vi "Simulation.vi"() -> ()   [LabVIEW 2011]
uses:
  Pumps_Valves_Dependencies_Global.vi
panel:
  out "Slide":dbl(slide) scale=0.0..100.0
  out "Supply feed  2":bool(c317)
  out "Pipe3":bool
  out "T-Pipe 2":bool
  out "Supply feed  2":bool(c317)
  out "Pipe5":bool
  out "Pipe4":bool
  out "Mains Water Supply":bool
  out "Pipe2":bool
  out "Supply feed":bool(c317)
  out "T-Pipe":bool
  out "Tank C":dbl(slide) scale=0.0..100.0
  out "Tank D":dbl(slide) scale=0.0..100.0
  out "Tank B":dbl(slide) scale=0.0..100.0
  out "Pipe":bool
  out "Pipe 1":bool
  out "Tank A":dbl(slide) scale=0.0..100.0
  out "Salt Saturator":dbl(slide) scale=0.0..100.0
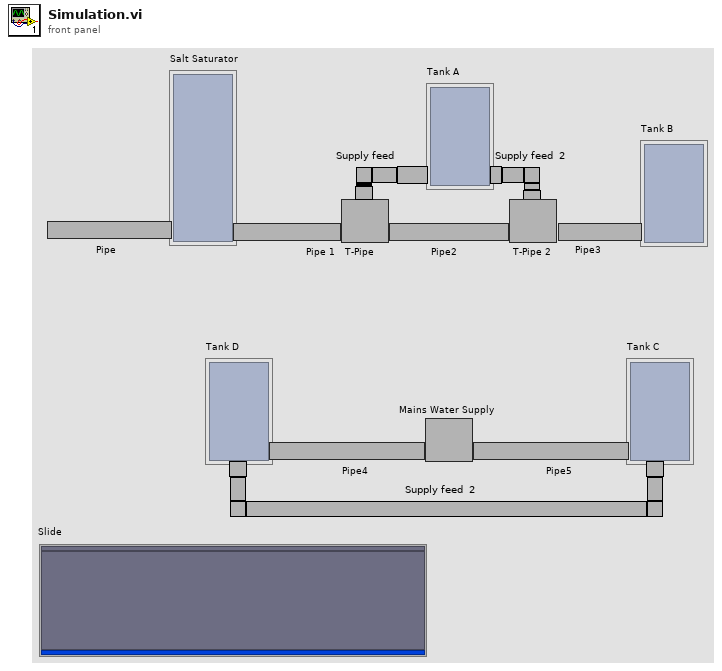
[diagram p1: front panel]
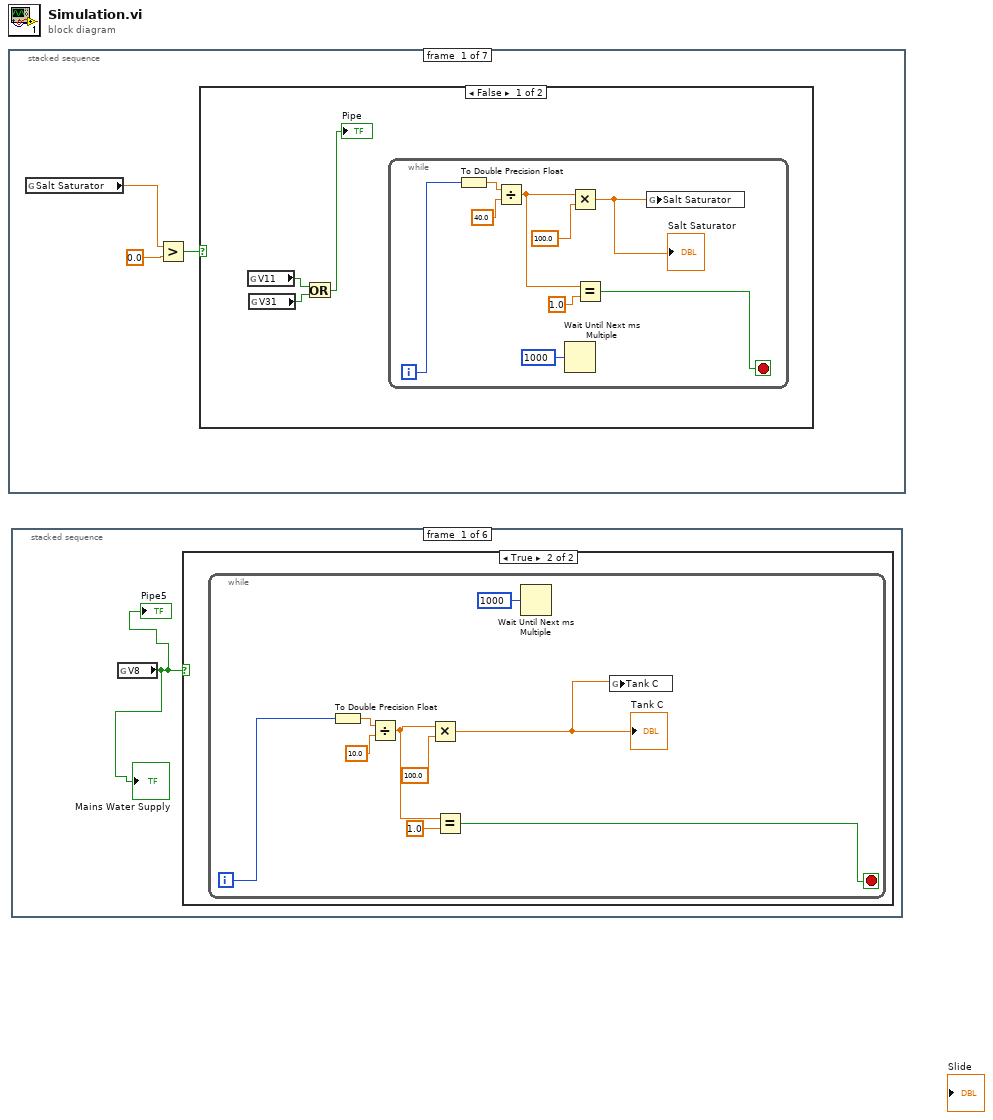
[diagram p0: block diagram]
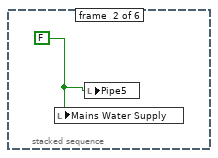
[diagram p3: hidden frame]
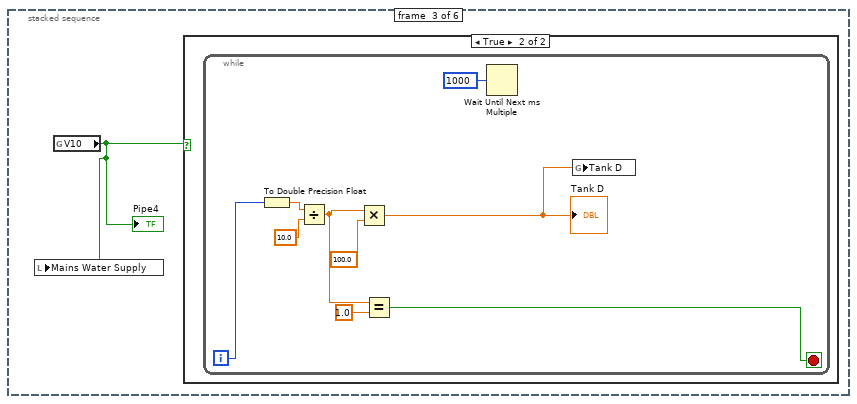
[diagram p4: hidden frame]
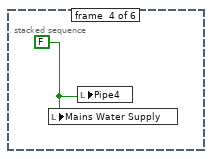
[diagram p6: hidden frame]
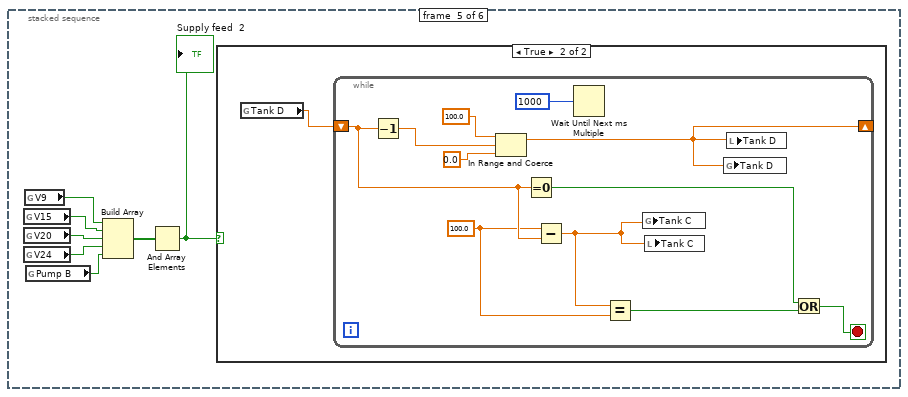
[diagram p7: hidden frame]
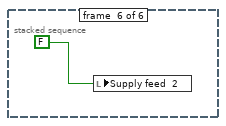
[diagram p9: hidden frame]
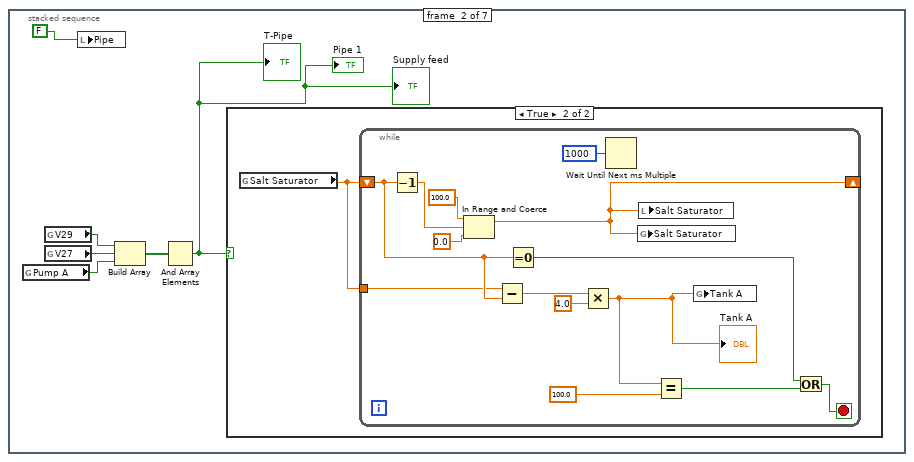
[diagram p11: hidden frame]
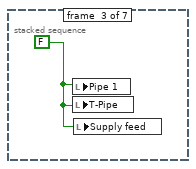
[diagram p13: hidden frame]
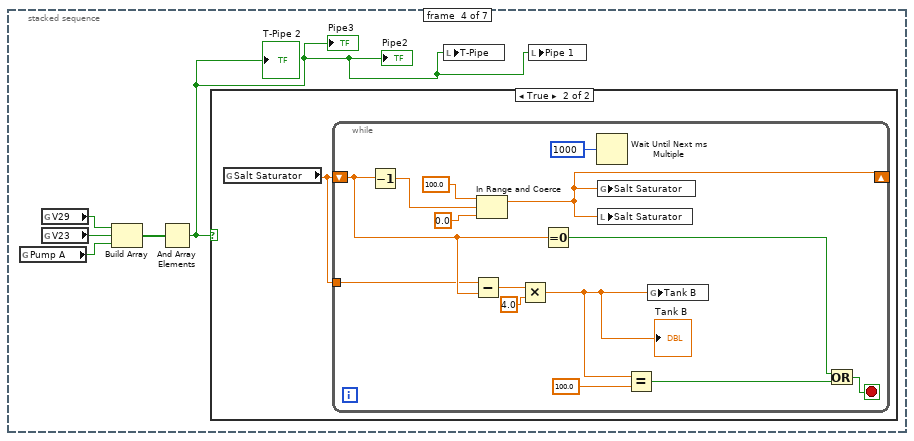
[diagram p14: hidden frame]
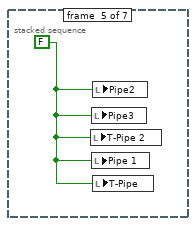
[diagram p16: hidden frame]
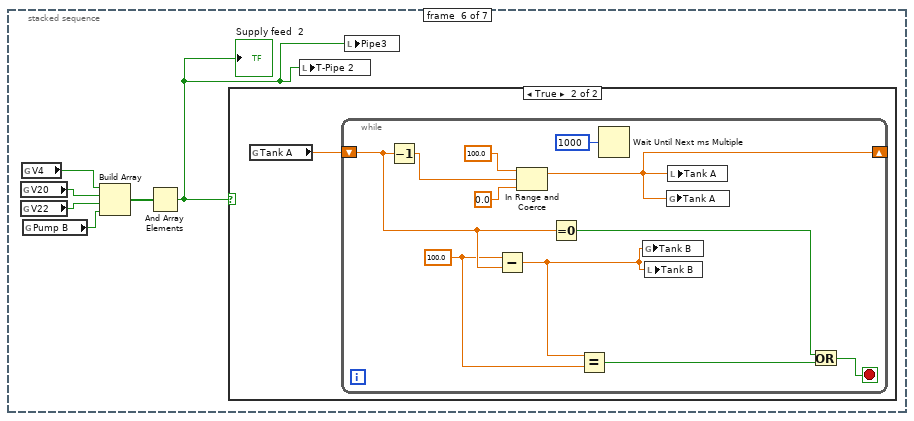
[diagram p17: hidden frame]
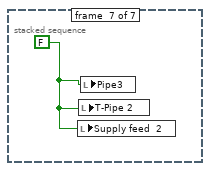
[diagram p19: hidden frame]
diagram:
  n1 = stacked-sequence {
    frame #0 {
      n2 = global read "Pumps_Valves_Dependencies_Global.vi" "Salt Saturator"() -> (w2:dbl)
      n3 = Greater?(x=w2, y=0.0) -> (0:w3:bool)
      n4 = case shown="False" w3 {
        frame False {
          n5 = global read "Pumps_Valves_Dependencies_Global.vi" "V11"() -> (w5:bool)
          n6 = global read "Pumps_Valves_Dependencies_Global.vi" "V31"() -> (w6:bool)
          n7 = Or(x=w5, y=w6) -> (x .or. y?=→"Pipe":bool)
          n8 = while {
            i -> [w7]
            stop <- w9 stop-if-true
            n9 = To Double Precision Float(number=w7) -> (double precision float=w11:dbl)
            n10 = Divide(x=w11, y=40.0) -> (x/y=w13:dbl)
            n11 = Wait Until Next ms Multiple(millisecond multiple=u32 1000) -> ()  [unwired: 1 out]
            n12 = Multiply(x=w13, y=100.0) -> (x*y=w8:dbl)
            "Salt Saturator" <- w8
            n13 = Equal?(x=w13, y=1.0) -> (x = y?=w9:bool)
            n14 = global write "Pumps_Valves_Dependencies_Global.vi" "Salt Saturator"(w8) -> ()
          }
        }
        frame True {
        }
      }
    }
    frame #1 {
      n15 = global read "Pumps_Valves_Dependencies_Global.vi" "Pump A"() -> (w19:bool)
      n16 = global read "Pumps_Valves_Dependencies_Global.vi" "V29"() -> (w17:bool)
      n17 = global read "Pumps_Valves_Dependencies_Global.vi" "V27"() -> (w18:bool)
      n18 = local write "Pipe"(FALSE) -> ()
      n19 = Build Array(w17, w18, w19) -> (w20:bool[])
      n20 = And Array Elements(Boolean array=w20) -> (logical AND=w16:bool)
      "Pipe 1" <- w16
      "T-Pipe" <- w16
      "Supply feed" <- w16
      n21 = case shown="True" w16 {
        frame False {
        }
        frame True {
          n22 = global read "Pumps_Valves_Dependencies_Global.vi" "Salt Saturator"() -> (w22:dbl)
          n23 = while {
            shift-right: [w30] -> _
            shift-left: w22 -> [w26]
            tunnel: w22 -> [w23]
            stop <- w34 stop-if-true
            n24 = Decrement(x=w26) -> (x-1=w31:dbl)
            n25 = In Range and Coerce(upper limit=100.0 ("x"), x=w31, lower limit=0.0 ("x")) -> (coerced(x)=w30:dbl)  [unwired: 1 out]
            n26 = Subtract(x=w23, y=w26) -> (x-y=w27:dbl)
            n27 = Equal To 0?(x=w26) -> (x = 0?=w35:bool)
            n28 = Multiply(x=w27, y=4.0) -> (x*y=w24:dbl)
            "Tank A" <- w24
            n29 = Wait Until Next ms Multiple(millisecond multiple=u32 1000) -> ()  [unwired: 1 out]
            n30 = global write "Pumps_Valves_Dependencies_Global.vi" "Salt Saturator"(w30) -> ()
            n31 = local write "Salt Saturator"(w30) -> ()
            n32 = Equal?(x=w24, y=100.0) -> (x = y?=w29:bool)
            n33 = global write "Pumps_Valves_Dependencies_Global.vi" "Tank A"(w24) -> ()
            n34 = Or(x=w35, y=w29) -> (x .or. y?=w34:bool)
          }
        }
      }
    }
    frame #2 {
      w37 = FALSE
      n35 = local write "Pipe 1"(w37) -> ()
      n36 = local write "T-Pipe"(w37) -> ()
      n37 = local write "Supply feed"(w37) -> ()
    }
    frame #3 {
      n38 = global read "Pumps_Valves_Dependencies_Global.vi" "Pump A"() -> (w41:bool)
      n39 = global read "Pumps_Valves_Dependencies_Global.vi" "V29"() -> (w39:bool)
      n40 = global read "Pumps_Valves_Dependencies_Global.vi" "V23"() -> (w40:bool)
      n41 = Build Array(w39, w40, w41) -> (w42:bool[])
      n42 = And Array Elements(Boolean array=w42) -> (logical AND=w38:bool)
      "Pipe2" <- w38
      "T-Pipe 2" <- w38
      "Pipe3" <- w38
      n43 = case shown="True" w38 {
        frame False {
        }
        frame True {
          n44 = global read "Pumps_Valves_Dependencies_Global.vi" "Salt Saturator"() -> (w43:dbl)
          n45 = while {
            shift-right: [w52] -> _
            shift-left: w43 -> [w49]
            tunnel: w43 -> [w45]
            stop <- w55 stop-if-true
            n46 = Decrement(x=w49) -> (x-1=w51:dbl)
            n47 = Subtract(x=w45, y=w49) -> (x-y=w47:dbl)
            n48 = In Range and Coerce(upper limit=100.0 ("x"), x=w51, lower limit=0.0 ("x")) -> (coerced(x)=w52:dbl)  [unwired: 1 out]
            n49 = Multiply(x=w47, y=4.0) -> (x*y=w46:dbl)
            "Tank B" <- w46
            n50 = Equal To 0?(x=w49) -> (x = 0?=w56:bool)
            n51 = Wait Until Next ms Multiple(millisecond multiple=u32 1000) -> ()  [unwired: 1 out]
            n52 = global write "Pumps_Valves_Dependencies_Global.vi" "Salt Saturator"(w52) -> ()
            n53 = local write "Salt Saturator"(w52) -> ()
            n54 = Equal?(x=w46, y=100.0 ("x")) -> (x = y?=w50:bool)
            n55 = global write "Pumps_Valves_Dependencies_Global.vi" "Tank B"(w46) -> ()
            n56 = Or(x=w56, y=w50) -> (x .or. y?=w55:bool)
          }
        }
      }
      n57 = local write "T-Pipe"(w38) -> ()
      n58 = local write "Pipe 1"(w38) -> ()
    }
    frame #4 {
      w58 = FALSE
      n59 = local write "T-Pipe 2"(w58) -> ()
      n60 = local write "Pipe3"(w58) -> ()
      n61 = local write "Pipe 1"(w58) -> ()
      n62 = local write "Pipe2"(w58) -> ()
      n63 = local write "T-Pipe"(w58) -> ()
    }
    frame #5 {
      n64 = global read "Pumps_Valves_Dependencies_Global.vi" "V20"() -> (w63:bool)
      n65 = global read "Pumps_Valves_Dependencies_Global.vi" "V22"() -> (w62:bool)
      n66 = global read "Pumps_Valves_Dependencies_Global.vi" "V4"() -> (w64:bool)
      n67 = global read "Pumps_Valves_Dependencies_Global.vi" "Pump B"() -> (w61:bool)
      n68 = Build Array(w64, w63, w62, w61) -> (w60:bool[])
      n69 = And Array Elements(Boolean array=w60) -> (logical AND=w59:bool)
      "Supply feed  2" <- w59
      n70 = case shown="True" w59 {
        frame False {
        }
        frame True {
          n71 = global read "Pumps_Valves_Dependencies_Global.vi" "Tank A"() -> (w65:dbl)
          n72 = while {
            shift-right: [w70] -> _
            shift-left: w65 -> [w68]
            stop <- w75 stop-if-true
            w67 = 100.0 ("y")
            n73 = Decrement(x=w68) -> (x-1=w71:dbl)
            n74 = Subtract(x=w67, y=w68) -> (x-y=w66:dbl)
            n75 = In Range and Coerce(upper limit=100.0 ("x"), x=w71, lower limit=0.0 ("x")) -> (coerced(x)=w70:dbl)  [unwired: 1 out]
            n76 = Equal To 0?(x=w68) -> (x = 0?=w74:bool)
            n77 = Equal?(x=w66, y=w67) -> (x = y?=w69:bool)
            n78 = Wait Until Next ms Multiple(millisecond multiple=u32 1000) -> ()  [unwired: 1 out]
            n79 = global write "Pumps_Valves_Dependencies_Global.vi" "Tank B"(w66) -> ()
            n80 = local write "Tank B"(w66) -> ()
            n81 = global write "Pumps_Valves_Dependencies_Global.vi" "Tank A"(w70) -> ()
            n82 = local write "Tank A"(w70) -> ()
            n83 = Or(x=w74, y=w69) -> (x .or. y?=w75:bool)
          }
        }
      }
      n84 = local write "T-Pipe 2"(w59) -> ()
      n85 = local write "Pipe3"(w59) -> ()
    }
    frame #6 {
      w77 = FALSE
      n86 = local write "Supply feed  2"(w77) -> ()
      n87 = local write "T-Pipe 2"(w77) -> ()
      n88 = local write "Pipe3"(w77) -> ()
    }
  }
  n89 = stacked-sequence {
    frame #0 {
      n90 = global read "Pumps_Valves_Dependencies_Global.vi" "V8"() -> (w78:bool)
      "Mains Water Supply" <- w78
      "Pipe5" <- w78
      n91 = case shown="True" w78 {
        frame False {
        }
        frame True {
          n92 = while {
            i -> [w80]
            stop <- w79 stop-if-true
            n93 = To Double Precision Float(number=w80) -> (double precision float=w85:dbl)
            n94 = Divide(x=w85, y=10.0) -> (x/y=w83:dbl)
            n95 = Multiply(x=w83, y=100.0) -> (x*y=w81:dbl)
            "Tank C" <- w81
            n96 = Equal?(x=w83, y=1.0) -> (x = y?=w79:bool)
            n97 = Wait Until Next ms Multiple(millisecond multiple=u32 1000) -> ()  [unwired: 1 out]
            n98 = global write "Pumps_Valves_Dependencies_Global.vi" "Tank C"(w81) -> ()
          }
        }
      }
    }
    frame #1 {
      w88 = FALSE
      n99 = local write "Mains Water Supply"(w88) -> ()
      n100 = local write "Pipe5"(w88) -> ()
    }
    frame #2 {
      n101 = global read "Pumps_Valves_Dependencies_Global.vi" "V10"() -> (w89:bool)
      "Pipe4" <- w89
      n102 = local write "Mains Water Supply"(w89) -> ()
      n103 = case shown="True" w89 {
        frame False {
        }
        frame True {
          n104 = while {
            i -> [w92]
            stop <- w91 stop-if-true
            n105 = To Double Precision Float(number=w92) -> (double precision float=w94:dbl)
            n106 = Divide(x=w94, y=10.0) -> (x/y=w96:dbl)
            n107 = Multiply(x=w96, y=100.0) -> (x*y=w90:dbl)
            "Tank D" <- w90
            n108 = Equal?(x=w96, y=1.0) -> (x = y?=w91:bool)
            n109 = Wait Until Next ms Multiple(millisecond multiple=u32 1000) -> ()  [unwired: 1 out]
            n110 = global write "Pumps_Valves_Dependencies_Global.vi" "Tank D"(w90) -> ()
          }
        }
      }
    }
    frame #3 {
      w99 = FALSE
      n111 = local write "Mains Water Supply"(w99) -> ()
      n112 = local write "Pipe4"(w99) -> ()
    }
    frame #4 {
      n113 = global read "Pumps_Valves_Dependencies_Global.vi" "V15"() -> (w102:bool)
      n114 = global read "Pumps_Valves_Dependencies_Global.vi" "V20"() -> (w103:bool)
      n115 = global read "Pumps_Valves_Dependencies_Global.vi" "V24"() -> (w104:bool)
      n116 = global read "Pumps_Valves_Dependencies_Global.vi" "V9"() -> (w101:bool)
      n117 = global read "Pumps_Valves_Dependencies_Global.vi" "Pump B"() -> (w105:bool)
      n118 = Build Array(w101, w102, w103, w104, w105) -> (w106:bool[])
      n119 = And Array Elements(Boolean array=w106) -> (logical AND=w100:bool)
      "Supply feed  2" <- w100
      n120 = case shown="True" w100 {
        frame False {
        }
        frame True {
          n121 = global read "Pumps_Valves_Dependencies_Global.vi" "Tank D"() -> (w107:dbl)
          n122 = while {
            shift-right: [w112] -> _
            shift-left: w107 -> [w111]
            stop <- w113 stop-if-true
            w110 = 100.0 ("y")
            n123 = Decrement(x=w111) -> (x-1=w115:dbl)
            n124 = In Range and Coerce(upper limit=100.0 ("x"), x=w115, lower limit=0.0 ("x")) -> (coerced(x)=w112:dbl)  [unwired: 1 out]
            n125 = Equal To 0?(x=w111) -> (x = 0?=w114:bool)
            n126 = Subtract(x=w110, y=w111) -> (x-y=w109:dbl)
            n127 = Wait Until Next ms Multiple(millisecond multiple=u32 1000) -> ()  [unwired: 1 out]
            n128 = Equal?(x=w109, y=w110) -> (x = y?=w108:bool)
            n129 = global write "Pumps_Valves_Dependencies_Global.vi" "Tank C"(w109) -> ()
            n130 = local write "Tank C"(w109) -> ()
            n131 = global write "Pumps_Valves_Dependencies_Global.vi" "Tank D"(w112) -> ()
            n132 = local write "Tank D"(w112) -> ()
            n133 = Or(x=w114, y=w108) -> (x .or. y?=w113:bool)
          }
        }
      }
    }
    frame #5 {
      n134 = local write "Supply feed  2"(FALSE) -> ()
    }
  }
